vi "WAIT_FOR_PID.vi"(10 "argv":string[](array[string]), 11 "args":u8) -> ()   [LabVIEW 2015]
uses:
  Team Code/Robot Global Data.vi
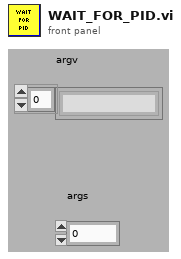
[diagram p1: front panel]
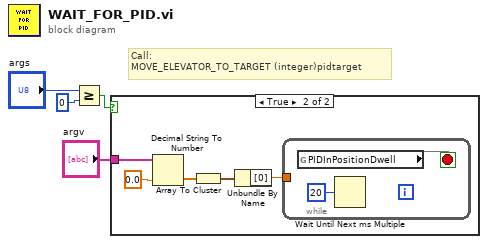
[diagram p0: block diagram]
diagram:
  # "Call:\nMOVE_ELEVATOR_TO_TARGET (integer)pidtarget"
  n1 = Greater Or Equal?(x="args", y=u8 0) -> (x >= y?=w4:bool)
  n2 = case shown="True" w4 {
    tunnel: "argv" -> [_ w9]
    frame False {
    }
    frame True {
      n3 = Decimal String To Number(string=w9, default (0L)=0.0 ("default (0 I32)")) -> (number=w7:dbl[])  [unwired: 2 out]
      n4 = Array To Cluster(array=w7) -> (cluster=w6:cluster{"[0]":dbl, "[1]":dbl})
      n5 = Unbundle By Name(w6) -> ("[0]"=w5:dbl)
      n6 = while {
        tunnel: w5 -> [_]
        stop <- w11 stop-if-true
        n7 = global read "Robot Global Data.vi" "PIDInPositionDwell"() -> (w11)
        n8 = Wait Until Next ms Multiple(millisecond multiple=u32 20) -> ()  [unwired: 1 out]
      }
    }
  }
